vi "Graph Sync.vi"(6 "Control Ref Queue":T1, 7 "Actual Transform In":T2, 8 "error in (no error)":errorcluster, 11 "3D Plot.lvclass in":refnum<class "3D Plot.lvclass">) -> (0 "error out":errorcluster, 3 "3D Plot.lvclass out":refnum<class "3D Plot.lvclass">, 5 "Actual Transform Out":T2)   [LabVIEW 2020, in "3D Plot.lvclass"]
uses:
  3D Plot.lvclass
  Actual Transform.ctl
  Range Clusters.ctl
  3DMathPlot Ctrl Act Queue.ctl
  3DMathPlot Ctrl Act Cluster.ctl
  3DMathPlot State Class.ctl
  3D Plot.lvclass/3D Plot.ctl
  NI_Math Plot Private Lib.lvlib
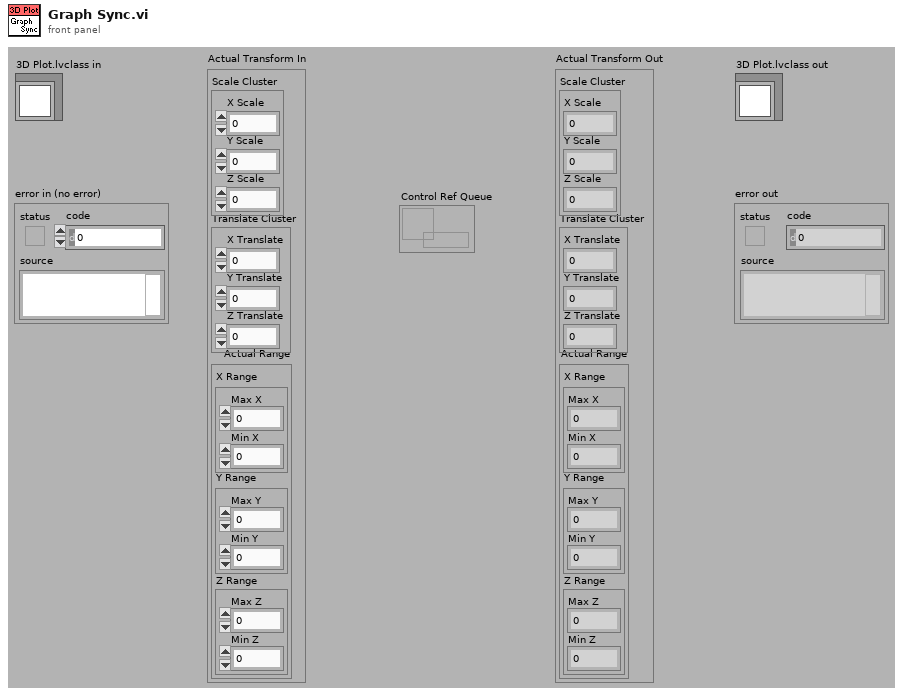
[diagram p1: front panel]
types:
  T1 = typedef "3DMathPlot Ctrl Act Queue.ctl" = refnum<queue>
  T2 = typedef "3D Plot.lvclass/Actual Transform.ctl" = cluster{"Scale Cluster":cluster{"X Scale":sgl, "Y Scale":sgl, "Z Scale":sgl}, "Translate Cluster":cluster{"X Translate":sgl, "Y Translate":sgl, "Z Translate":sgl}, "Actual Range":T3}
  T3 = typedef "3D Plot.lvclass/Range Clusters.ctl" = cluster{"X Range":cluster{"Max X":sgl, "Min X":sgl}, "Y Range":cluster{"Max Y":sgl, "Min Y":sgl}, "Z Range":cluster{"Max Z":sgl, "Min Z":sgl}}
  T4 = enum32{"Towards X-Y Plane", "Towards X-Z Plane", "Towards Y-Z Plane", "User Defined"}
  T5 = typedef "3D Plot.lvclass/Caption Property.ctl" = cluster{"Show Caption":cluster{"Show Normal X Caption":bool, "Show Normal Y Caption":bool, "Show Normal Z Caption":bool, "Show Opposite X Caption":bool, "Show Opposite Y Caption":bool, "Show Opposite Z Caption":bool}, "Caption Color":cluster{"Caption Color X":u32, "Caption Color Y":u32, "Caption Color Z":u32}, "Caption Size":cluster{"Caption Size X":u16, "Caption Size Y":u16, "Caption Size Z":u16}, "Caption String":cluster{"Caption X":string, "Caption Y":string, "Caption Z ":string}}
  T6 = typedef "3D Plot.lvclass/Label Property.ctl" = cluster{"Show Label":cluster{"Show Normal X Label":bool, "Show Normal Y Label":bool, "Show Normal Z Label":bool, "Show Opposite X Label":bool, "Show Opposite Y Label":bool, "Show Opposite Z Label":bool}, "Label Color":cluster{"Label Color X":u32, "Label Color Y":u32, "Label Color Z":u32}, "Label Size":cluster{"Label Size X":u16, "Label Size Y":u16, "Labe Size Z":u16}}
  T7 = typedef "3D Plot.lvclass/Format Property.ctl" = string[]
  T8 = typedef "3D Plot.lvclass/Range Property.ctl" = cluster{"Range Cluster":T3, "Auto Range":cluster{"Auto Range X":bool, "Auto Range Y":bool, "Auto Range Z":bool}, "Inverted":cluster{"Inverted X":bool, "Inverted Y":bool, "Inverted Z":bool}, "Logarithm":cluster{"Logarithm X":bool, "Logarithm Y":bool, "Logarithm Z":bool}}
  T9 = cluster{"Major Count X":u16, "Major Count Y":u16, "Major Count Z":u16}
  T10 = typedef "3D Plot.lvclass/Value Pair Property.ctl" = T11[]
  T11 = typedef "3D Plot.lvclass/Value Pair Cluster.ctl" = cluster{"Value Pair Array":cluster{"Value":sgl, "Name":string}[], "Show Tick":bool, "Show Grid":bool, " Label Mode":enum16{"Name", "Value", "None"}}
  T12 = typedef "3DMathPlot Ctrl Act Cluster.ctl" = cluster{"3D Picture Control":refnum<vi>, "Render Window Refnum":refnum<vi>, "XY Graph":refnum<vi>, "Intensity Graph":refnum<vi>, "Color Legend Palette":refnum<vi>, "Projection Palette":refnum<vi>, "XControl  Ref":refnum<vi>, "Facade Ref":refnum<vi>, "Export Image Ref":refnum<vi>, "Clear Data Flag":bool, "Display State Change Class":T13}
  T13 = typedef "3DMathPlot State Class.ctl" = enum16{"Update All Objects (Undo)", "Update Light Object Only", "Update Axis Object Only", "Update Plot Object Only", "Update Cursor Object Only", "Update Axis Plot Cursor Objects", "No Update"}
  T14 = typedef "LVRectTypeDef.ctl" = cluster{"Left":i16, "Top":i16, "Right":i16, "Bottom":i16}
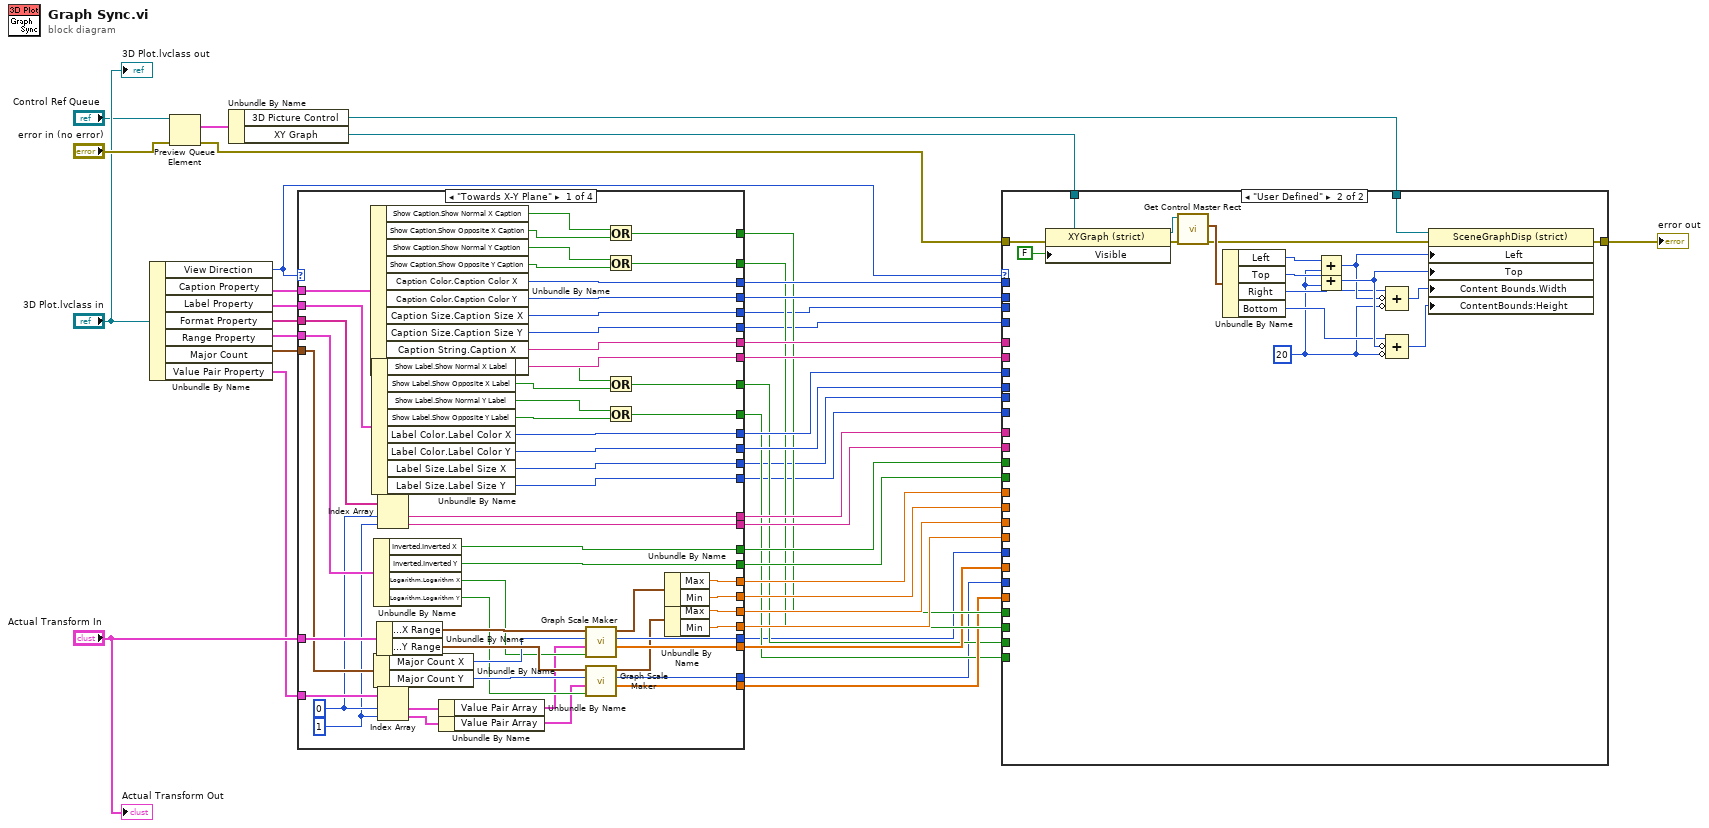
[diagram p0: block diagram]
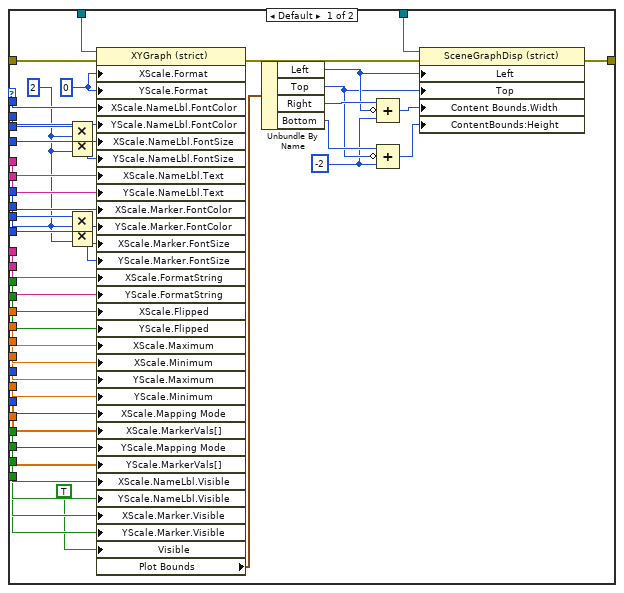
[diagram p2: hidden frame]
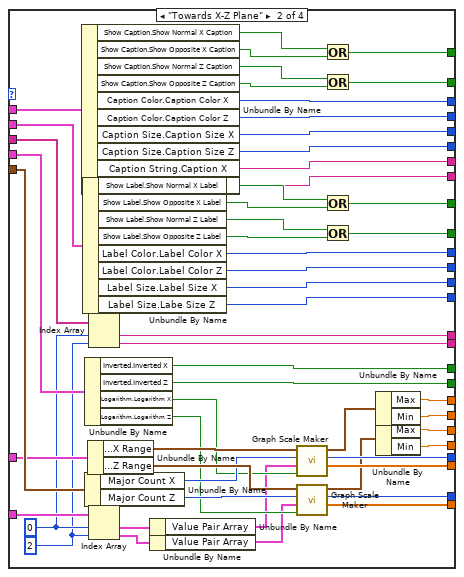
[diagram p3: hidden frame]
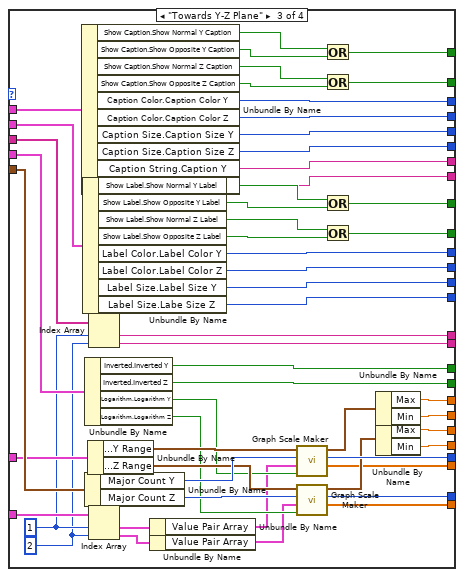
[diagram p4: hidden frame]
diagram:
  n1 = Unbundle By Name("3D Plot.lvclass in") -> ("View Direction"=w9:T4, "Caption Property"=w13:T5, "Label Property"=w12:T6, "Format Property"=w7:T7, "Range Property"=w11:T8, "Major Count"=w10:T9, "Value Pair Property"=w8:T10)
  n2 = Preview Queue Element(queue="Control Ref Queue", error in (no error)="error in (no error)") -> (element=w3:T12, error out=w2:errorcluster)  [unwired: 3 out]
  n3 = Unbundle By Name(w3) -> ("3D Picture Control"=w4:refnum<vi>, "XY Graph"=w1:refnum<vi>)
  n4 = case shown="\"Towards X-Y Plane\"" w9 {
    tunnel: w13 -> [w97 w144 w199 _]
    tunnel: [w96 w137 w193 _] -> w37
    tunnel: [w95 w136 w192 _] -> w36
    tunnel: [w94 w135 w191 _] -> w17
    tunnel: [w93 w134 w190 _] -> w16
    tunnel: [w92 w132 w188 _] -> w35
    tunnel: [w91 w133 w189 _] -> w34
    tunnel: w12 -> [w90 w143 w198 _]
    tunnel: w11 -> [w89 w142 w175 _]
    tunnel: [w88 w124 w180 _] -> w33
    tunnel: [w87 w125 w181 _] -> w32
    tunnel: [w57 w111 w166 _] -> w31
    tunnel: [w56 w110 w165 _] -> w30
    tunnel: [w54 w109 w164 _] -> w29
    tunnel: [w53 w108 w163 _] -> w28
    tunnel: [w86 w129 w185 _] -> w27
    tunnel: [w85 w128 w183 _] -> w26
    tunnel: [w84 w127 w184 _] -> w15
    tunnel: [w83 w126 w182 _] -> w14
    tunnel: [w44 w99 w155 _] -> w25
    tunnel: [w43 w98 w156 _] -> w24
    tunnel: [w80 w139 w195 _] -> w23
    tunnel: [w77 w138 w194 _] -> w22
    tunnel: "Actual Transform In" -> [w76 w140 w196 _]
    tunnel: w10 -> [w75 w141 w197 _]
    tunnel: w8 -> [w50 w105 w162 _]
    tunnel: [w60 w114 w167 _] -> w21
    tunnel: [w59 w113 w168 _] -> w20
    tunnel: [w70 w130 w186 _] -> w19
    tunnel: [w69 w131 w187 _] -> w18
    tunnel: w7 -> [w47 w102 w157 _]
    tunnel: [w64 w119 w174 _] -> w6
    tunnel: [w63 w118 w173 _] -> w5
    frame "Towards X-Y Plane" {
      w45 = 1 ("index")
      w46 = 0 ("index")
      n5 = Unbundle By Name(w97) -> ("Show Caption.Show Normal X Caption"=w82:bool, "Show Caption.Show Opposite X Caption"=w81:bool, "Show Caption.Show Normal Y Caption"=w79:bool, "Show Caption.Show Opposite Y Caption"=w78:bool, "Caption Color.Caption Color X"=w96:u32, "Caption Color.Caption Color Y"=w95:u32, "Caption Size.Caption Size X"=w94:u16, "Caption Size.Caption Size Y"=w93:u16, "Caption String.Caption X"=w91:string, "Caption String.Caption Y"=w92:string)
      n6 = Unbundle By Name(w90) -> ("Show Label.Show Normal X Label"=w74:bool, "Show Label.Show Opposite X Label"=w73:bool, "Show Label.Show Normal Y Label"=w72:bool, "Show Label.Show Opposite Y Label"=w71:bool, "Label Color.Label Color X"=w86:u32, "Label Color.Label Color Y"=w85:u32, "Label Size.Label Size X"=w84:u16, "Label Size.Label Size Y"=w83:u16)
      n7 = Unbundle By Name(w89) -> ("Inverted.Inverted X"=w88:bool, "Inverted.Inverted Y"=w87:bool, "Logarithm.Logarithm X"=w62:bool, "Logarithm.Logarithm Y"=w61:bool)
      n8 = Unbundle By Name(w75) -> ("Major Count X"=w65:u16, "Major Count Y"=w67:u16)
      n9 = Unbundle By Name(w76) -> ("Actual Range.X Range"=w66:cluster{"Max X":sgl, "Min X":sgl}, "Actual Range.Y Range"=w68:cluster{"Max Y":sgl, "Min Y":sgl})
      n10 = Index Array(array=w47, index #1=w46, index #2=w45) -> (element #1=w44:string, element #2=w43:string)
      n11 = Index Array(array=w50, index #1=w46, index #2=w45) -> (element #1=w52:T11, element #2=w51:T11)
      n12 = Unbundle By Name(w52) -> ("Value Pair Array"=w49:cluster{"Value":sgl, "Name":string}[])
      n13 = Unbundle By Name(w51) -> ("Value Pair Array"=w48:cluster{"Value":sgl, "Name":string}[])
      n14 = call "Graph Scale Maker.vi"("Logarithm?"=w62, "Value Pair Info Array"=w49, "Major Ticks"=w65, "Range In"=w66) -> ("Maker Array"=w60:sgl[], "Mapping Mode"=w64:u8, "Range Out"=w58:cluster{"Max":sgl, "Min":sgl})  [unwired: 5 out]
      n15 = call "Graph Scale Maker.vi"("Logarithm?"=w61, "Value Pair Info Array"=w48, "Major Ticks"=w67, "Range In"=w68) -> ("Maker Array"=w59:sgl[], "Mapping Mode"=w63:u8, "Range Out"=w55:cluster{"Max":sgl, "Min":sgl})  [unwired: 5 out]
      n16 = Or(x=w82, y=w81) -> (x .or. y?=w80:bool)
      n17 = Or(x=w79, y=w78) -> (x .or. y?=w77:bool)
      n18 = Or(x=w74, y=w73) -> (x .or. y?=w69:bool)
      n19 = Or(x=w72, y=w71) -> (x .or. y?=w70:bool)
      n20 = Unbundle By Name(w58) -> ("Max"=w57:sgl, "Min"=w56:sgl)
      n21 = Unbundle By Name(w55) -> ("Max"=w54:sgl, "Min"=w53:sgl)
    }
    frame "Towards X-Z Plane" {
      w100 = 2 ("index")
      w101 = 0 ("index")
      n22 = Unbundle By Name(w144) -> ("Show Caption.Show Normal X Caption"=w152:bool, "Show Caption.Show Opposite X Caption"=w151:bool, "Show Caption.Show Normal Z Caption"=w150:bool, "Show Caption.Show Opposite Z Caption"=w149:bool, "Caption Color.Caption Color X"=w137:u32, "Caption Color.Caption Color Z"=w136:u32, "Caption Size.Caption Size X"=w135:u16, "Caption Size.Caption Size Z"=w134:u16, "Caption String.Caption X"=w133:string, "Caption String.Caption Z"=w132:string)
      n23 = Unbundle By Name(w143) -> ("Show Label.Show Normal X Label"=w148:bool, "Show Label.Show Opposite X Label"=w147:bool, "Show Label.Show Normal Z Label"=w146:bool, "Show Label.Show Opposite Z Label"=w145:bool, "Label Color.Label Color X"=w129:u32, "Label Color.Label Color Z"=w128:u32, "Label Size.Label Size X"=w127:u16, "Label Size.Labe Size Z"=w126:u16)
      n24 = Unbundle By Name(w142) -> ("Inverted.Inverted X"=w124:bool, "Inverted.Inverted Z"=w125:bool, "Logarithm.Logarithm X"=w117:bool, "Logarithm.Logarithm Z"=w116:bool)
      n25 = Unbundle By Name(w141) -> ("Major Count X"=w120:u16, "Major Count Z"=w122:u16)
      n26 = Unbundle By Name(w140) -> ("Actual Range.X Range"=w121:cluster{"Max X":sgl, "Min X":sgl}, "Actual Range.Z Range"=w123:cluster{"Max Z":sgl, "Min Z":sgl})
      n27 = Index Array(array=w102, index #1=w101, index #2=w100) -> (element #1=w99:string, element #2=w98:string)
      n28 = Index Array(array=w105, index #1=w101, index #2=w100) -> (element #1=w107:T11, element #2=w106:T11)
      n29 = Unbundle By Name(w107) -> ("Value Pair Array"=w104:cluster{"Value":sgl, "Name":string}[])
      n30 = Unbundle By Name(w106) -> ("Value Pair Array"=w103:cluster{"Value":sgl, "Name":string}[])
      n31 = call "Graph Scale Maker.vi"("Logarithm?"=w117, "Value Pair Info Array"=w104, "Major Ticks"=w120, "Range In"=w121) -> ("Maker Array"=w114:sgl[], "Mapping Mode"=w119:u8, "Range Out"=w115:cluster{"Max":sgl, "Min":sgl})  [unwired: 5 out]
      n32 = call "Graph Scale Maker.vi"("Logarithm?"=w116, "Value Pair Info Array"=w103, "Major Ticks"=w122, "Range In"=w123) -> ("Maker Array"=w113:sgl[], "Mapping Mode"=w118:u8, "Range Out"=w112:cluster{"Max":sgl, "Min":sgl})  [unwired: 5 out]
      n33 = Or(x=w152, y=w151) -> (x .or. y?=w139:bool)
      n34 = Or(x=w150, y=w149) -> (x .or. y?=w138:bool)
      n35 = Or(x=w148, y=w147) -> (x .or. y?=w131:bool)
      n36 = Or(x=w146, y=w145) -> (x .or. y?=w130:bool)
      n37 = Unbundle By Name(w115) -> ("Max"=w111:sgl, "Min"=w110:sgl)
      n38 = Unbundle By Name(w112) -> ("Max"=w109:sgl, "Min"=w108:sgl)
    }
    frame "Towards Y-Z Plane" {
      w153 = 2 ("index")
      w154 = 1 ("index")
      n39 = Unbundle By Name(w199) -> ("Show Caption.Show Normal Y Caption"=w207:bool, "Show Caption.Show Opposite Y Caption"=w206:bool, "Show Caption.Show Normal Z Caption"=w205:bool, "Show Caption.Show Opposite Z Caption"=w204:bool, "Caption Color.Caption Color Y"=w193:u32, "Caption Color.Caption Color Z"=w192:u32, "Caption Size.Caption Size Y"=w191:u16, "Caption Size.Caption Size Z"=w190:u16, "Caption String.Caption Y"=w189:string, "Caption String.Caption Z"=w188:string)
      n40 = Unbundle By Name(w198) -> ("Show Label.Show Normal Y Label"=w203:bool, "Show Label.Show Opposite Y Label"=w202:bool, "Show Label.Show Normal Z Label"=w201:bool, "Show Label.Show Opposite Z Label"=w200:bool, "Label Color.Label Color Y"=w185:u32, "Label Color.Label Color Z"=w183:u32, "Label Size.Label Size Y"=w184:u16, "Label Size.Labe Size Z"=w182:u16)
      n41 = Unbundle By Name(w175) -> ("Inverted.Inverted Y"=w180:bool, "Inverted.Inverted Z"=w181:bool, "Logarithm.Logarithm Y"=w172:bool, "Logarithm.Logarithm Z"=w171:bool)
      n42 = Unbundle By Name(w197) -> ("Major Count Y"=w178:u16, "Major Count Z"=w176:u16)
      n43 = Unbundle By Name(w196) -> ("Actual Range.Y Range"=w179:cluster{"Max Y":sgl, "Min Y":sgl}, "Actual Range.Z Range"=w177:cluster{"Max Z":sgl, "Min Z":sgl})
      n44 = Index Array(array=w157, index #1=w154, index #2=w153) -> (element #1=w155:string, element #2=w156:string)
      n45 = Index Array(array=w162, index #1=w154, index #2=w153) -> (element #1=w161:T11, element #2=w159:T11)
      n46 = Unbundle By Name(w161) -> ("Value Pair Array"=w160:cluster{"Value":sgl, "Name":string}[])
      n47 = Unbundle By Name(w159) -> ("Value Pair Array"=w158:cluster{"Value":sgl, "Name":string}[])
      n48 = call "Graph Scale Maker.vi"("Logarithm?"=w172, "Value Pair Info Array"=w160, "Major Ticks"=w178, "Range In"=w179) -> ("Maker Array"=w167:sgl[], "Mapping Mode"=w174:u8, "Range Out"=w170:cluster{"Max":sgl, "Min":sgl})  [unwired: 5 out]
      n49 = call "Graph Scale Maker.vi"("Logarithm?"=w171, "Value Pair Info Array"=w158, "Major Ticks"=w176, "Range In"=w177) -> ("Maker Array"=w168:sgl[], "Mapping Mode"=w173:u8, "Range Out"=w169:cluster{"Max":sgl, "Min":sgl})  [unwired: 5 out]
      n50 = Or(x=w207, y=w206) -> (x .or. y?=w195:bool)
      n51 = Or(x=w205, y=w204) -> (x .or. y?=w194:bool)
      n52 = Or(x=w203, y=w202) -> (x .or. y?=w187:bool)
      n53 = Or(x=w201, y=w200) -> (x .or. y?=w186:bool)
      n54 = Unbundle By Name(w170) -> ("Max"=w166:sgl, "Min"=w165:sgl)
      n55 = Unbundle By Name(w169) -> ("Max"=w164:sgl, "Min"=w163:sgl)
    }
    frame "User Defined" {
    }
  }
  n56 = case shown="\"User Defined\"" w9 {
    tunnel: w37 -> [w253 _]
    tunnel: w36 -> [w252 _]
    tunnel: w35 -> [w251 _]
    tunnel: w34 -> [w250 _]
    tunnel: w33 -> [w249 _]
    tunnel: w32 -> [w248 _]
    tunnel: w31 -> [w247 _]
    tunnel: w30 -> [w246 _]
    tunnel: w29 -> [w245 _]
    tunnel: w28 -> [w244 _]
    tunnel: w27 -> [w243 _]
    tunnel: w26 -> [w242 _]
    tunnel: w1 -> [w241 w271]
    tunnel: w25 -> [w239 _]
    tunnel: w24 -> [w238 _]
    tunnel: w23 -> [w228 _]
    tunnel: w22 -> [w227 _]
    tunnel: w21 -> [w215 _]
    tunnel: w20 -> [w216 _]
    tunnel: w19 -> [w225 _]
    tunnel: w18 -> [w226 _]
    tunnel: w17 -> [w233 _]
    tunnel: w16 -> [w232 _]
    tunnel: w15 -> [w231 _]
    tunnel: w14 -> [w230 _]
    tunnel: w2 -> [w224 w269]
    tunnel: [w218 w259] -> w42
    tunnel: w4 -> [w220 w260]
    tunnel: w6 -> [w214 _]
    tunnel: w5 -> [w213 _]
    frame Default {
      w208 = i16 -2
      w229 = u16 2
      w240 = u8 0 ("X Scale.Display Format:Precision")
      n57 = Multiply(x=w233, y=w229) -> (x*y=w237:u16)
      n58 = Multiply(x=w232, y=w229) -> (x*y=w236:u16)
      n59 = Multiply(x=w231, y=w229) -> (x*y=w235:u16)
      n60 = Multiply(x=w230, y=w229) -> (x*y=w234:u16)
      n61 = property class="XYGraph (strict)"(reference=w241, error in=w224, "XScale.Format"=w240, "YScale.Format"=w240, "XScale.NameLbl.FontColor"=w253, "YScale.NameLbl.FontColor"=w252, "XScale.NameLbl.FontSize"=w237, "YScale.NameLbl.FontSize"=w236, "XScale.NameLbl.Text"=w250, "YScale.NameLbl.Text"=w251, "XScale.Marker.FontColor"=w243, "YScale.Marker.FontColor"=w242, "XScale.Marker.FontSize"=w235, "YScale.Marker.FontSize"=w234, "XScale.FormatString"=w239, "YScale.FormatString"=w238, "XScale.Flipped"=w249, "YScale.Flipped"=w248, "XScale.Maximum"=w247, "XScale.Minimum"=w246, "YScale.Maximum"=w245, "YScale.Minimum"=w244, "XScale.Mapping Mode"=w214, "XScale.MarkerVals[]"=w215, "YScale.Mapping Mode"=w213, "YScale.MarkerVals[]"=w216, "XScale.NameLbl.Visible"=w228, "YScale.NameLbl.Visible"=w227, "XScale.Marker.Visible"=w226, "YScale.Marker.Visible"=w225, "Visible"=TRUE ("X Scale.Visible")) -> (error out=w219:errorcluster, "Plot Bounds"=w217:T14)  [unwired: 1 out]
      n62 = Unbundle By Name(w217) -> ("Left"=w212:i16, "Top"=w211:i16, "Right"=w222:i16, "Bottom"=w221:i16)
      n63 = Compound Arithmetic op=ADD(w222, invert w212, w208) -> (w210:i16)
      n64 = Compound Arithmetic op=ADD(w221, invert w211, w208) -> (w209:i16)
      n65 = property class="SceneGraphDisp (strict)"(reference=w220, error in=w219, "Left"=w212, "Top"=w211, "Content Bounds.Width"=w210, "ContentBounds:Height"=w209) -> (error out=w218:errorcluster)  [unwired: 1 out]
    }
    frame "User Defined" {
      w258 = i16 20 ("y")
      n66 = property class="XYGraph (strict)"(reference=w271, error in=w269, "Visible"=FALSE) -> (reference out=w257:refnum<vi>, error out=w255:errorcluster)
      n67 = call "Get Control Master Rect.vi"("error in (no error)"=w255, "reference"=w257) -> ("error out"=w254:errorcluster, "Master Bounds Rect"=w256:T14)  [unwired: 8 out]
      n68 = Unbundle By Name(w256) -> ("Left"=w262:i16, "Top"=w263:i16, "Right"=w261:i16, "Bottom"=w265:i16)
      n69 = Add(x=w262, y=w258) -> (x+y=w264:i16)
      n70 = Add(x=w263, y=w258) -> (x+y=w266:i16)
      n71 = Compound Arithmetic op=ADD(w261, invert w264, invert w258) -> (w268:i16)
      n72 = Compound Arithmetic op=ADD(w265, invert w266, invert w258) -> (w267:i16)
      n73 = property class="SceneGraphDisp (strict)"(reference=w260, error in=w254, "Left"=w264, "Top"=w266, "Content Bounds.Width"=w268, "ContentBounds:Height"=w267) -> (error out=w259:errorcluster)  [unwired: 1 out]
    }
  }
  "error out" <- w42
  "3D Plot.lvclass out" <- "3D Plot.lvclass in"
  "Actual Transform Out" <- "Actual Transform In"
